vi "Merge Data.vi"(8 "error in":errorcluster, 10 "Analyzed":refnum<class "Instrument.lvclass">, 11 "Acquired":refnum<class "CRDS.lvclass">) -> (0 "error out":errorcluster, 3 "CRDS out":refnum<class "CRDS.lvclass">)   [LabVIEW 2015, in "CRDS.lvclass"]
doc: "The VI Merge Data is used strictly here to merge the serial data with the rest of the data. THIS VI WILL BE NO LONGER NECESSARY WHEN ISSUES RELATING TO RT EXE ARE FIXED!!"
uses:
  CRDS.lvclass
  Instrument/Instrument.lvclass
  CRDS.lvclass/CRDS.ctl
  Cell/CRDS Cell.lvclass/CRDS Cell.ctl
  Data/Cell/CRDS Cell Data.lvclass/CRDS Cell Data.ctl
  Cell/Read Data.vi
  Data/Cell/Read extParam.vi
  Data/Cell/Write extParam.vi
  Cell/Write Data.vi
  Cell/Read corr tau0.vi
  Cell/Read tau_0.vi
  Cell/Write corr tau0.vi
  Cell/Write tau_0.vi
  Data/Cell/CRDS Cell Data.lvclass
  Data/Main/CRDS Data.lvclass
  Cell/CRDS Cell.lvclass
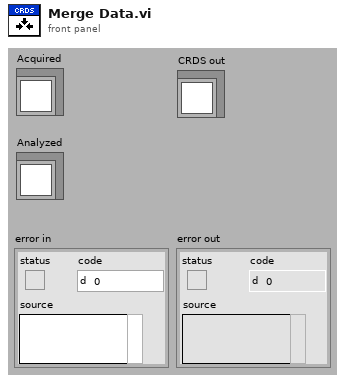
[diagram p1: front panel]
types:
  T1 = typedef "extparam.ctl" = cluster{"Tau":sgl, "Tau0cor":sgl, "ext":sgl, "extCorr":sgl, "stdevTau":sgl, "eTau":sgl, "taucorr":sgl, "Tau0":sgl, "max":sgl}
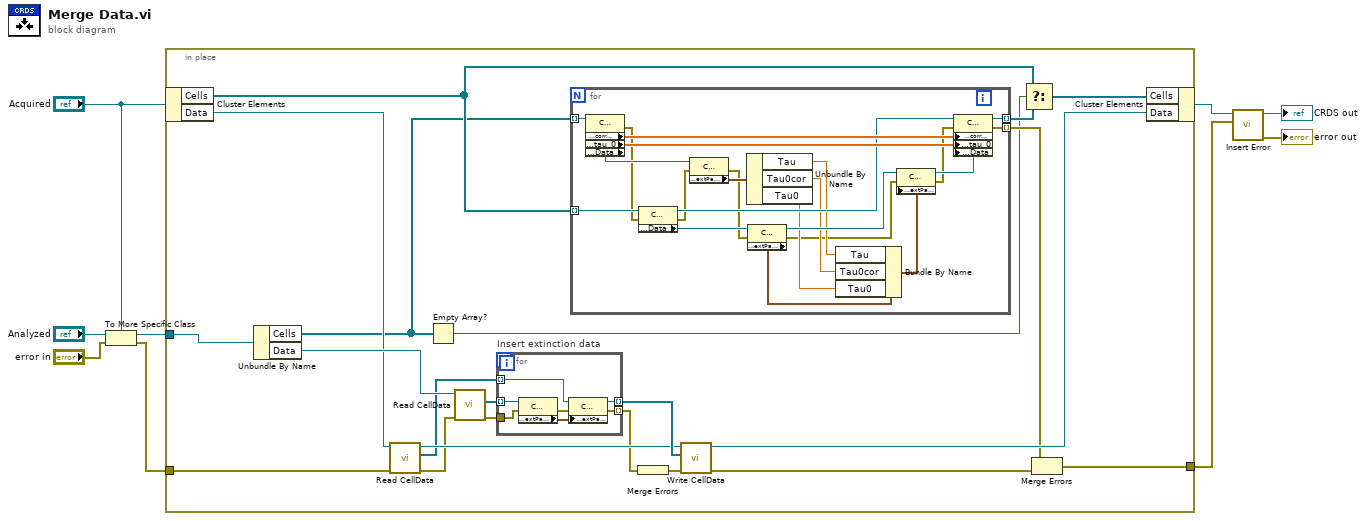
[diagram p0: block diagram]
diagram:
  n1 = To More Specific Class(target class="Acquired", reference="Analyzed", error in="error in") -> (specific class reference=w5:refnum<class "CRDS.lvclass">, error out=w6:errorcluster)
  n2 = in-place {
    in-place-border: w6 -> [w27]
    in-place-border: w5 -> [w30]
    in-place-border: [w12] -> w1
    n3 = in-place-cluster #1("Acquired") -> ("Cells"=w23:refnum<class "CRDS Cell.lvclass">[], "Data"=w26:refnum<class "CRDS Data.lvclass">)
    n4 = Unbundle By Name(w30) -> ("Cells"=w11:refnum<class "CRDS Cell.lvclass">[], "Data"=w29:refnum<class "CRDS Data.lvclass">)
    n5 = call "Read CellData.vi"("error in"=w27, "CRDS Data in"=w26) -> ("error out"=w19:errorcluster, "CellData"=w17:refnum<class "CRDS Cell Data.lvclass">[], "CRDS Data out"=w20:refnum<class "CRDS Data.lvclass">)  [unwired: 7 in]
    n6 = Empty Array?(array=w11) -> (empty?=w10:bool)
    n7 = call "Read CellData.vi"("error in"=w19, "CRDS Data in"=w29) -> ("error out"=w22:errorcluster, "CellData"=w18:refnum<class "CRDS Cell Data.lvclass">[])  [unwired: 7 in, 1 out]
    n8 = for "Insert extinction data" {
      tunnel: w18 -> [w59] mode=indexing
      tunnel: w22 -> [w58]
      tunnel: w17 -> [w55] mode=indexing
      tunnel: [w54] -> w16 mode=indexing
      tunnel: [w53] -> w21 mode=indexing
      n9 = property class="CRDS Cell"(reference=w59, error in=w58) -> (error out=w56:errorcluster, "Data Access:extParam"=w57:T1)  [unwired: 1 out]
      n10 = property class="CRDS Cell"(reference=w55, error in=w56, "Data Access:extParam"=w57) -> (reference out=w53:refnum<class "CRDS Cell Data.lvclass">, error out=w54:errorcluster)
    }
    n11 = for {
      tunnel: w11 -> [w52] mode=indexing
      tunnel: w23 -> [w47] mode=indexing
      tunnel: [w49] -> w25 mode=indexing
      tunnel: [w37] -> w14 mode=indexing
      n12 = property class="CRDS Cell"(reference=w52) -> (error out=w36:errorcluster, "Data Access:corr tau0"=w51:dbl[], "Data Access:tau_0"=w50:dbl[], "Data Access:Data"=w48:refnum<class "CRDS Cell Data.lvclass">)  [unwired: 1 in, 1 out]
      n13 = property class="CRDS Cell"(reference=w47, error in=w36) -> (reference out=w46:refnum<class "CRDS Cell.lvclass">, error out=w35:errorcluster, "Data Access:Data"=w45:refnum<class "CRDS Cell Data.lvclass">)
      n14 = property class="CRDS Cell"(reference=w48, error in=w35) -> (error out=w34:errorcluster, "Data Access:extParam"=w42:T1)  [unwired: 1 out]
      n15 = Unbundle By Name(w42) -> ("Tau"=w33:sgl, "Tau0cor"=w41:sgl, "Tau0"=w40:sgl)
      n16 = property class="CRDS Cell"(reference=w45, error in=w34) -> (reference out=w43:refnum<class "CRDS Cell Data.lvclass">, error out=w32:errorcluster, "Data Access:extParam"=w44:T1)
      n17 = Bundle By Name(cluster=w44, "Tau"=w33, "Tau0cor"=w41, "Tau0"=w40) -> (w39:T1)
      n18 = property class="CRDS Cell"(reference=w43, error in=w32, "Data Access:extParam"=w39) -> (reference out=w38:refnum<class "CRDS Cell Data.lvclass">, error out=w31:errorcluster)
      n19 = property class="CRDS Cell"(reference=w46, error in=w31, "Data Access:corr tau0"=w51, "Data Access:tau_0"=w50, "Data Access:Data"=w38) -> (reference out=w49:refnum<class "CRDS Cell.lvclass">, error out=w37:errorcluster)
    }
    n20 = Merge Errors(w16) -> (w15:errorcluster)
    n21 = call "Write CellData.vi"("error in"=w15, "CellData"=w21, "CRDS Data in"=w20) -> ("error out"=w13:errorcluster, "CRDS Data out"=w28:refnum<class "CRDS Data.lvclass">)  [unwired: 7 in]
    n22 = Select(t=w23, s=w10, f=w25) -> (s? t:f=w24:refnum<class "CRDS Cell.lvclass">[])
    n23 = Merge Errors(w14, w13) -> (w12:errorcluster)
    n24 = in-place-cluster #1("Cells"=w24, "Data"=w28) -> (w4:refnum<class "CRDS.lvclass">)
  }
  n25 = call "Insert Error.vi"("err"=w1, "Instrument in"=w4) -> ("error out"=→"error out":errorcluster, "Instrument out"=→"CRDS out":refnum<class "CRDS.lvclass">)  [unwired: 7 in, 1 out]
